vi "Main Engine All Engine Reference Close.vi"(8 "error in":errorcluster, 11 "Data Cluster":T1={"IP Address"="", "Hardware Info"=[], "Main Engine Response Q"=refnum, "Bin File Refnum"=refnum, "TCP Engine Response Q"=refnum, "TCP Engine Refnum"=refnum, "DAQ Device Info"=[], "Serial Device Info"=[], "Hardware Info Notifier"=refnum, "Main Engine Command Q"=refnum, "Variant Data"=variant, "Engine Name"="Slot5_6551_AO", "Interface"="AO", "SubCmd"="", "Serial Mode"="", "Serial Engine Reference"=[], "PLL Locked?"=FALSE, "PLL Status"="", "Ethernet Mode"=0, "Eth TCP Engine Ref"=[], "Ethernet IP Address"=[], "CPU Load"=FALSE, "Sys Session "="", "Sys Ref"=refnum, "Current time"=timestamp(0 s since 1904-01-01), "CPU Frequency"=0.0, "RT-All Q Ref"=[], "DAQ-Engine Ref"=[], "Main Engine Logging File Path"=path ""} {"Hardware Info"."Is Present?" items=["Initializing"=-2, "Unknown"=-1, "Not Present"=0, "Present"=1]}) -> (0 "error out":errorcluster)   [LabVIEW 2021]
doc: "All Rights Reserved © 2023 SyncSols"
uses:
  Controls/Main Engine State Machine Data Cluster.ctl
  Controls/Main Engine Hardware Info Data Cluster.ctl
  Controls/Main Engine DAQ Device Info.ctl
  Controls/Main Engine Serial Card Details.ctl
  Controls/Main Engine Hardware Loop Data.ctl
  Controls/Main Engine Command Cluster.ctl
  Controls/Main Engine TCP Command Data.ctl
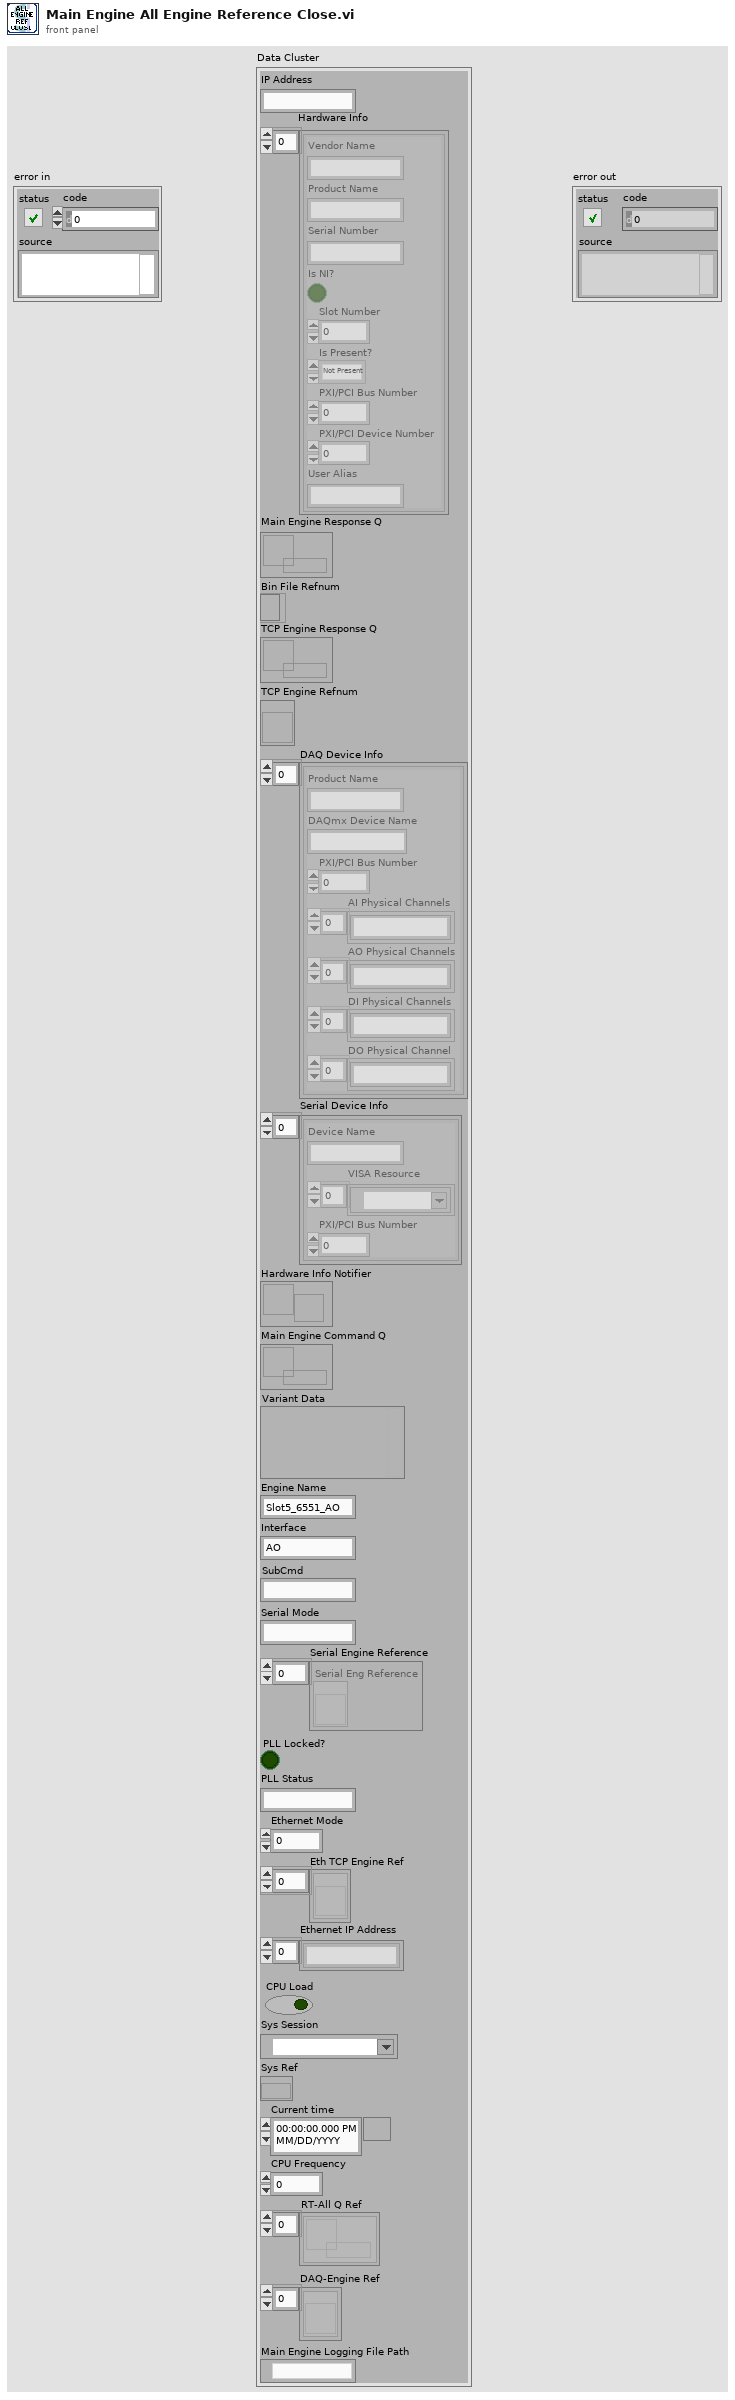
[diagram p1: front panel]
types:
  T1 = typedef "Main Engine State Machine Data Cluster.ctl" = cluster{"IP Address":string, "Hardware Info":T2[], "Main Engine Response Q":refnum<queue>, "Bin File Refnum":refnum<file>, "TCP Engine Response Q":refnum<queue>, "TCP Engine Refnum":refnum<vi>, "DAQ Device Info":T3[], "Serial Device Info":T4[], "Hardware Info Notifier":refnum<notifier>, "Main Engine Command Q":refnum<queue>, "Variant Data":variant, "Engine Name":string, "Interface":string, "SubCmd":string, "Serial Mode":string, "Serial Engine Reference":refnum<vi>[], "PLL Locked?":bool, "PLL Status":string, "Ethernet Mode":u8, "Eth TCP Engine Ref":refnum<vi>[], "Ethernet IP Address":string[], "CPU Load":bool, "Sys Session ":refnum<k21>, "Sys Ref":refnum<k20>, "Current time":timestamp, "CPU Frequency":dbl, "RT-All Q Ref":refnum<queue>[], "DAQ-Engine Ref":refnum<vi>[], "Main Engine Logging File Path":path}
  T2 = typedef "Main Engine Hardware Info Data Cluster.ctl" = cluster{"Vendor Name":string, "Product Name":string, "Serial Number":string, "Is NI?":bool, "Slot Number":i32, "Is Present?":i32, "PXI/PCI Bus Number":u32, "PXI/PCI Device Number":u32, "User Alias":string}
  T3 = typedef "Main Engine DAQ Device Info.ctl" = cluster{"Product Name":string, "DAQmx Device Name":string, "PXI/PCI Bus Number":u32, "AI Physical Channels":string[], "AO Physical Channels":string[], "DI Physical Channels":string[], "DO Physical Channel":string[]}
  T4 = typedef "Main Engine Serial Card Details.ctl" = cluster{"Device Name":string, "VISA Resource":refnum<visa-resource-name>[], "PXI/PCI Bus Number":u32}
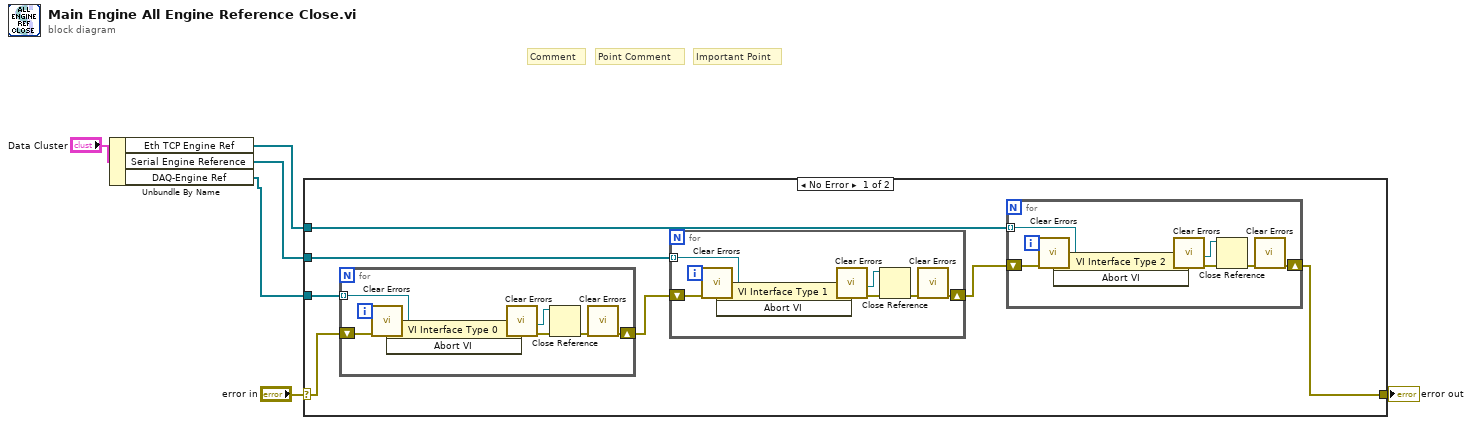
[diagram p0: block diagram]
diagram:
  # "Important Point"
  # "Point Comment"
  # "Comment"
  n1 = Unbundle By Name("Data Cluster") -> ("Eth TCP Engine Ref"=w3:refnum<vi>[], "Serial Engine Reference"=w2:refnum<vi>[], "DAQ-Engine Ref"=w1:refnum<vi>[])
  n2 = case shown="No Error" "error in" {
    selector: "error in" -> [w12 w38]
    tunnel: [w7 w38] -> w6
    tunnel: w1 -> [w13 _]
    tunnel: w2 -> [w10 _]
    tunnel: w3 -> [w9 _]
    frame No Error {
      n3 = for {
        tunnel: w13 -> [w36] mode=indexing
        shift-right: [w30] -> w11
        shift-left: w12 -> [w32]
        n4 = call <vilib>:"Clear Errors.vi"("error in (no error)"=w32) -> ("error out"=w31:errorcluster)  [unwired: 5 in, 1 out]
        n5 = invoke class="VI Interface Type 0" method="Abort VI"(reference=w36, error in=w31) -> (reference out=w34:refnum<vi>, error out=w35:errorcluster)  [unwired: 1 in, 1 out]
        n6 = call <vilib>:"Clear Errors.vi"("error in (no error)"=w35) -> ("error out"=w33:errorcluster)  [unwired: 5 in, 1 out]
        n7 = Close Reference(reference=w34, error in (no error)=w33) -> (error out=w37:errorcluster)
        n8 = call <vilib>:"Clear Errors.vi"("error in (no error)"=w37) -> ("error out"=w30:errorcluster)  [unwired: 5 in, 1 out]
      }
      n9 = for {
        tunnel: w10 -> [w28] mode=indexing
        shift-right: [w22] -> w8
        shift-left: w11 -> [w24]
        n10 = call <vilib>:"Clear Errors.vi"("error in (no error)"=w24) -> ("error out"=w23:errorcluster)  [unwired: 5 in, 1 out]
        n11 = invoke class="VI Interface Type 1" method="Abort VI"(reference=w28, error in=w23) -> (reference out=w26:refnum<vi>, error out=w27:errorcluster)  [unwired: 1 in, 1 out]
        n12 = call <vilib>:"Clear Errors.vi"("error in (no error)"=w27) -> ("error out"=w25:errorcluster)  [unwired: 5 in, 1 out]
        n13 = Close Reference(reference=w26, error in (no error)=w25) -> (error out=w29:errorcluster)
        n14 = call <vilib>:"Clear Errors.vi"("error in (no error)"=w29) -> ("error out"=w22:errorcluster)  [unwired: 5 in, 1 out]
      }
      n15 = for {
        tunnel: w9 -> [w20] mode=indexing
        shift-right: [w14] -> w7
        shift-left: w8 -> [w16]
        n16 = call <vilib>:"Clear Errors.vi"("error in (no error)"=w16) -> ("error out"=w15:errorcluster)  [unwired: 5 in, 1 out]
        n17 = invoke class="VI Interface Type 2" method="Abort VI"(reference=w20, error in=w15) -> (reference out=w18:refnum<vi>, error out=w19:errorcluster)  [unwired: 1 in, 1 out]
        n18 = call <vilib>:"Clear Errors.vi"("error in (no error)"=w19) -> ("error out"=w17:errorcluster)  [unwired: 5 in, 1 out]
        n19 = Close Reference(reference=w18, error in (no error)=w17) -> (error out=w21:errorcluster)
        n20 = call <vilib>:"Clear Errors.vi"("error in (no error)"=w21) -> ("error out"=w14:errorcluster)  [unwired: 5 in, 1 out]
      }
    }
    frame Error {
    }
  }
  "error out" <- w6
